vi "add_range_DC_check_to_report.vi"(8 "error in (no error)":errorcluster, 11 "Boc12 in":refnum<class "Boc12.lvclass">) -> (0 "error out":errorcluster, 3 "Boc12 out":refnum<class "Boc12.lvclass">)   [LabVIEW 2017, in "Boc12.lvclass"]
uses:
  Boc12.lvclass
  Report.lvclass/Report.ctl
  <vilib>/Utility/NIReport.llb/Append Text Table to Report (wrap).vi
  <vilib>/Utility/NIReport.llb/NI_report.lvclass
  Report.lvclass
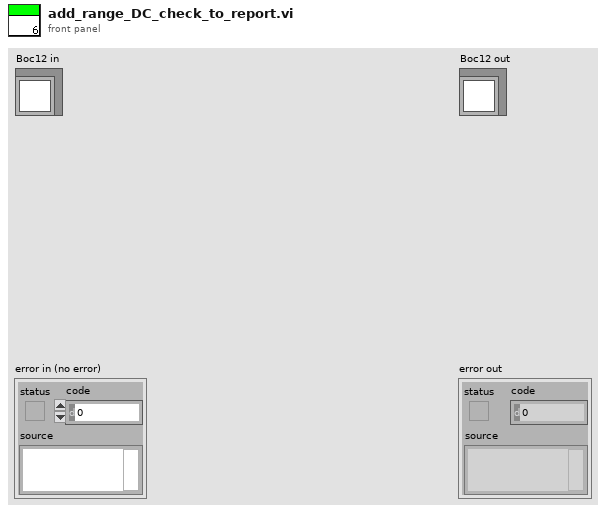
[diagram p1: front panel]
types:
  T1 = cluster{"position (excel)":cluster{"row":i32, "column":i32}, "name (excel)":string, "bookmark (word)":string}
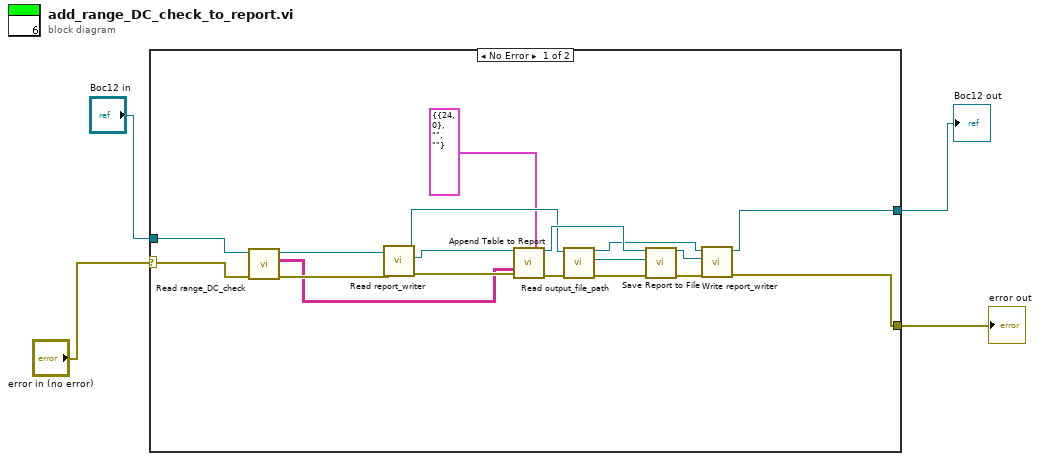
[diagram p0: block diagram]
diagram:
  n1 = case shown="No Error" "error in (no error)" {
    selector: "error in (no error)" -> [w21 w23]
    tunnel: "Boc12 in" -> [w22 w24]
    tunnel: [w7 w24] -> w2
    tunnel: [w6 w23] -> w1
    frame No Error {
      n2 = call-dynamic "Read range_DC_check.vi"("error in (no error)"=w21, "Report in"=w22) -> ("error out"=w9:errorcluster, "range_DC_check"=w8:string[][], "Report out"=w10:refnum<class "Boc12.lvclass">)  [unwired: 7 in]
      n3 = call "Read report_writer.vi"("error in (no error)"=w9, "Report in"=w10) -> ("error out"=w18:errorcluster, "NI_report.lvclass"=w19:refnum<class "NI_report.lvclass">, "Report out"=w15:refnum<class "Boc12.lvclass">)  [unwired: 7 in]
      n4 = call-poly <vilib>:"Append Table to Report.vi"("report in"=w19, "MS Office parameters"=T1 {"position (excel)"={"row"=24, "column"=0}, "name (excel)"="", "bookmark (word)"=""}, "text data"=w8, "error in (no error)"=w18) -> ("report out"=w20:refnum<class "NI_report.lvclass">, "error out"=w16:errorcluster)  [unwired: 8 in, 2 out]
      n5 = call "Read output_file_path.vi"("error in (no error)"=w16, "Report in"=w15) -> ("error out"=w17:errorcluster, "output_file_path"=w11:path, "Report out"=w12:refnum<class "Boc12.lvclass">)  [unwired: 7 in]
      n6 = call-dynamic "Save Report to File.vi"("report in"=w20, "report file path"=w11, "error in (no error)"=w17) -> ("report out"=w13:refnum<class "NI_report.lvclass">, "error out"=w14:errorcluster)  [unwired: 11 in]
      n7 = call "Write report_writer.vi"("error in (no error)"=w14, "NI_report.lvclass"=w13, "Report in"=w12) -> ("error out"=w6:errorcluster, "Report out"=w7:refnum<class "Boc12.lvclass">)  [unwired: 7 in]
    }
    frame Error {
    }
  }
  "error out" <- w1
  "Boc12 out" <- w2
